vi "Read Channel Setting.vi"(8 "error in (no error)":errorcluster, 11 "Channel configuration in":refnum<class "Channel configuration.lvclass">) -> (0 "error out":errorcluster, 2 "Channel Setting":T1={"Address"="None", "SW Alias"="127.0.0.1", "Description"="", "Enabled"=TRUE, "Type"="Type = Class \n"}, 3 "Channel configuration out":refnum<class "Channel configuration.lvclass">)   [LabVIEW 2025, in "Abstract Engine.lvlib" / "Channel configuration.lvclass"]
uses:
  Channel configuration.lvclass
  Default Channel.ctl
  Channel configuration.lvclass/Channel configuration.ctl
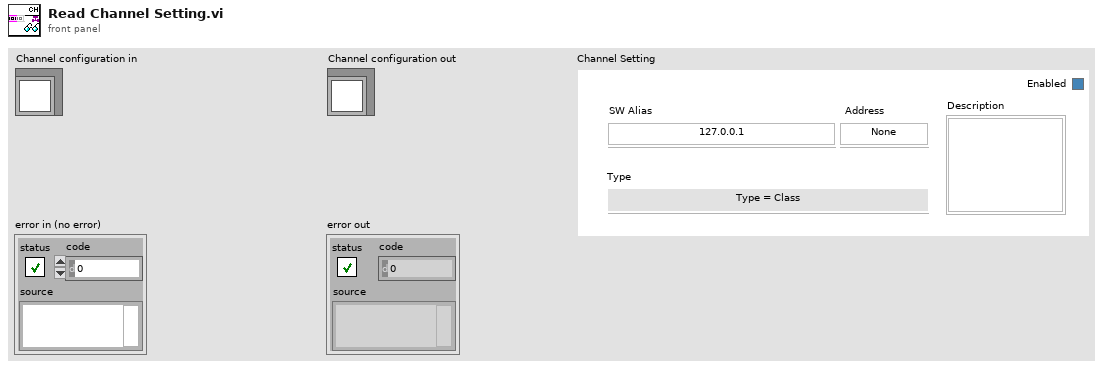
[diagram p1: front panel]
types:
  T1 = typedef "Abstract Engine.lvlib/Channel configuration.lvclass/Default Channel.ctl" = cluster{"Address":string, "SW Alias":string, "Description":string, "Enabled":bool, "Type":string}
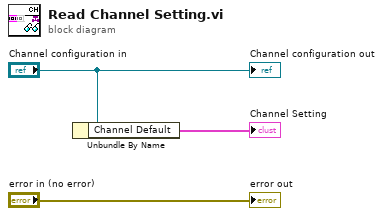
[diagram p0: block diagram]
diagram:
  n1 = Unbundle By Name("Channel configuration in") -> ("Channel Default"=→"Channel Setting":T1)
  "error out" <- "error in (no error)"
  "Channel configuration out" <- "Channel configuration in"
